vi "svx_Continuous Swept-Sine Prefix.vi"(8 "initial freq [Hz]":dbl, 9 "Fs":dbl, 10 "block size [samples]":i32, 11 "prefix len [samples]":i32) -> (1 "sin(x)":dbl[](array[numeric]), 2 "block size out [samples]":i32, 3 "prefix len out [samples]":i32)   [LabVIEW 2017]
uses:
  <vilib>/Analysis/1siggen.llb/Ramp Pattern by Samples.vi
  <vilib>/Analysis/NI_AALBase.lvlib
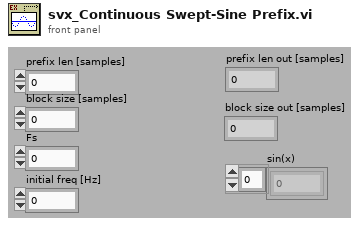
[diagram p1: front panel]
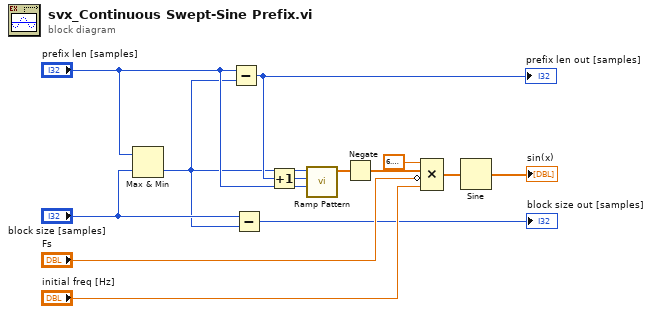
[diagram p0: block diagram]
diagram:
  n1 = Max & Min(x="prefix len [samples]", y="block size [samples]") -> (min(x,y)=w2:i32)  [unwired: 1 out]
  n2 = Subtract(x="prefix len [samples]", y=w2) -> (x-y=w13:i32)
  "prefix len out [samples]" <- w13
  n3 = Subtract(x="block size [samples]", y=w2) -> (x-y=→"block size out [samples]":i32)
  n4 = Increment(x=w13) -> (x+1=w12:i32)
  n5 = call-poly <vilib>:"Ramp Pattern.vi"("start"="prefix len [samples]", "end"=w12, "samples"=w2) -> ("Ramp Pattern"=w10:dbl[])  [unwired: 7 in, 1 out]
  n6 = Negate(x=w10) -> (-x=w9:dbl[])
  n7 = Compound Arithmetic op=MULTIPLY(6.283185307179586, w9, invert "Fs", "initial freq [Hz]") -> (w6:dbl[])
  n8 = Sine(x=w6) -> (sin(x)=→"sin(x)":dbl[])
